vi "MRayTurretHome.vi"(7 "Left to right":bool, 9 "Home volt":dbl, 10 "Volt at start":dbl, 11 "Turret POT volt":dbl) -> (2 "Turret Output":dbl)   [LabVIEW 2011]
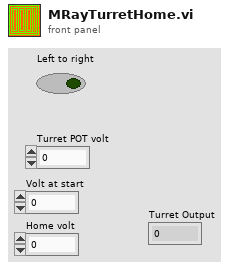
[diagram p1: front panel]
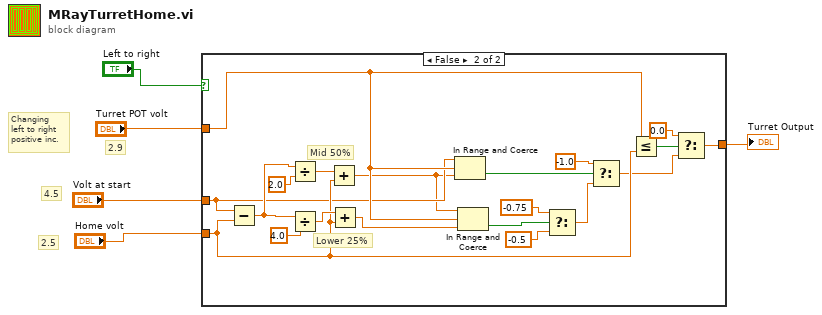
[diagram p0: block diagram]
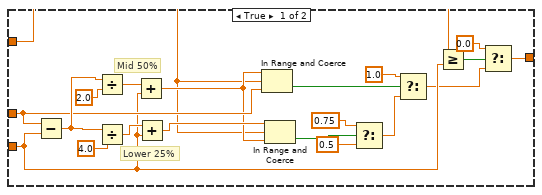
[diagram p2: hidden frame]
diagram:
  # "2.9"
  # "2.5"
  # "4.5"
  # "Changing\nleft to right\npositive inc."
  n1 = case shown="False" "Left to right" {
    tunnel: "Home volt" -> [w14 w35]
    tunnel: "Volt at start" -> [w17 w28]
    tunnel: "Turret POT volt" -> [w11 w34]
    tunnel: [w23 w43] -> w1
    frame True {
      # "Mid 50%"
      # "Lower 25%"
      n2 = Subtract(x=w17, y=w14) -> (x-y=w20:dbl)
      n3 = Divide(x=w20, y=2.0) -> (x/y=w19:dbl)
      n4 = Divide(x=w20, y=4.0) -> (x/y=w18:dbl)
      n5 = Add(x=w19, y=w14) -> (x+y=w12:dbl)
      n6 = Add(x=w18, y=w14) -> (x+y=w13:dbl)
      n7 = In Range and Coerce(upper limit=w12, x=w11, lower limit=w17) -> (In Range?=w16:bool)  [unwired: 1 out]
      n8 = In Range and Coerce(upper limit=w13, x=w11, lower limit=w12) -> (In Range?=w10:bool)  [unwired: 1 out]
      n9 = Select(t=0.75, s=w10, f=0.5) -> (s? t:f=w9:dbl)
      n10 = Select(t=1.0, s=w16, f=w9) -> (s? t:f=w6:dbl)
      n11 = Greater Or Equal?(x=w11, y=w14) -> (x >= y?=w25:bool)
      n12 = Select(t=0.0, s=w25, f=w6) -> (s? t:f=w23:dbl)
    }
    frame False {
      # "Mid 50%"
      # "Lower 25%"
      n13 = Subtract(x=w28, y=w35) -> (x-y=w40:dbl)
      n14 = Divide(x=w40, y=2.0) -> (x/y=w39:dbl)
      n15 = Divide(x=w40, y=4.0) -> (x/y=w38:dbl)
      n16 = Add(x=w39, y=w35) -> (x+y=w27:dbl)
      n17 = Add(x=w38, y=w35) -> (x+y=w26:dbl)
      n18 = In Range and Coerce(upper limit=w28, x=w34, lower limit=w27) -> (In Range?=w37:bool)  [unwired: 1 out]
      n19 = In Range and Coerce(upper limit=w27, x=w34, lower limit=w26) -> (In Range?=w33:bool)  [unwired: 1 out]
      n20 = Select(t=-0.75, s=w33, f=-0.5) -> (s? t:f=w32:dbl)
      n21 = Select(t=-1.0, s=w37, f=w32) -> (s? t:f=w29:dbl)
      n22 = Less Or Equal?(x=w34, y=w35) -> (x <= y?=w45:bool)
      n23 = Select(t=0.0, s=w45, f=w29) -> (s? t:f=w43:dbl)
    }
  }
  "Turret Output" <- w1
